vi "Parse Analyzer Results.vi"(6 "Fails":i32[](array[numeric]), 8 "error in":errorcluster, 9 "Passes":i32[](array[numeric]), 10 "VI Paths":path[](array[path]), 11 "Peer Review in":refnum<class "Peer Review.lvclass">) -> (0 "error out":errorcluster, 3 "Peer Review out":refnum<class "Peer Review.lvclass">)   [LabVIEW 2020, in "Peer Review.lvclass"]
uses:
  Peer Review.lvclass
  <vilib>/Utility/miscctls.llb/LVRowAndColumnUnsignedTypeDef.ctl
  Peer Review.lvclass/Peer Review.ctl
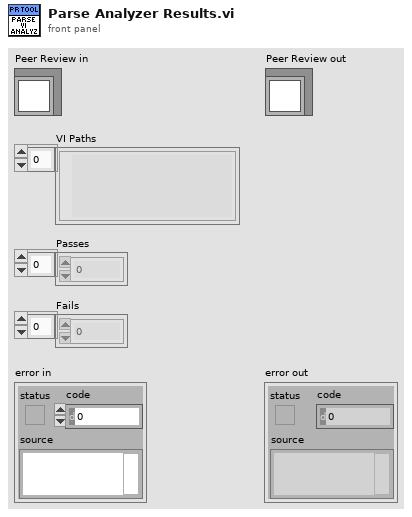
[diagram p1: front panel]
types:
  T1 = typedef "LVRowAndColumnUnsignedTypeDef.ctl" = cluster{"Row":u32, "Column":u32}
  T2 = typedef "Peer Review.lvclass/File Info.ctl" = cluster{"File ID":i32, "Commit ID":i32, "Reviewed Hash":string, "Relative Path":string, "File Path":path, "File Checksum":string, "State":T3, "FP Changes":i32, "BD Changes":i32, "FP Bounds Error":dbl, "BD Bounds Error":dbl, "Lines Added":i32, "Lines Removed":i32, "Analysis Passes":i32, "Analysis Fails":i32, "Attribute Changes":i32, "Reentrancy State":string, "Cyclomatic Complexity":i32, "Node Count":i32, "Revision Number":u32, "LabVIEW Version":string, "Description":string, "Master Path":path, "Master Checksum":string, "VI Type":T4, "LabVIEW File":bool, "Review Complete":bool, "File Ref":refnum<vi>}
  T3 = typedef "Peer Review.lvclass/File State.ctl" = enum16{"Interrogation Needed", "Modified", "Deleted", "Added", "Matches Previous", "No Changes", "Moved"}
  T4 = typedef "Peer Review.lvclass/VI Type.ctl" = enum32{"invalid VI type", "Standard VI", "Control VI", "Global VI", "Polymorphic VI", "Configuration VI", "SubSystem", "Facade VI", "Method VI", "Statechart Diagram VI"}
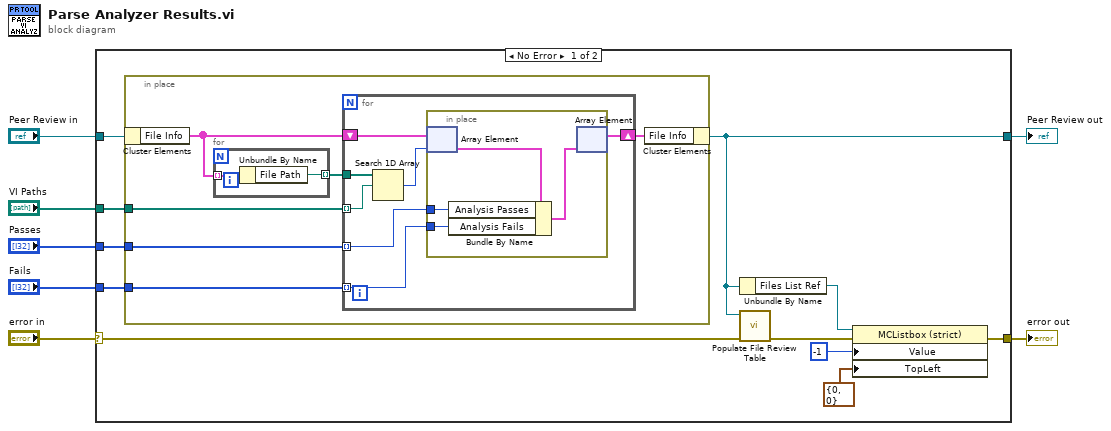
[diagram p0: block diagram]
diagram:
  n1 = case shown="No Error" "error in" {
    selector: "error in" -> [w18 w39]
    tunnel: [w14 w39] -> w6
    tunnel: [w8 w38] -> w4
    tunnel: "Peer Review in" -> [w9 w38]
    tunnel: "VI Paths" -> [w13 _]
    tunnel: "Passes" -> [w12 _]
    tunnel: "Fails" -> [w11 _]
    frame No Error {
      n2 = in-place {
        in-place-border: w13 -> [w23]
        in-place-border: w12 -> [w22]
        in-place-border: w11 -> [w21]
        n3 = in-place-cluster #1(w9) -> ("File Info"=w20:T2[])
        n4 = for {
          tunnel: w20 -> [w26] mode=indexing
          tunnel: [w25] -> w24 mode=indexing
          n5 = Unbundle By Name(w26) -> ("File Path"=w25:path)
        }
        n6 = for {
          tunnel: w24 -> [w33]
          shift-right: [w30] -> w19
          shift-left: w20 -> [w32]
          tunnel: w23 -> [w29] mode=indexing
          tunnel: w22 -> [w28] mode=indexing
          tunnel: w21 -> [w27] mode=indexing
          n7 = Search 1D Array(1D array=w33, element=w29) -> (index of element=w31:i32)  [unwired: 1 in]
          n8 = in-place "In Place Element Structure" {
            in-place-border: w28 -> [w36]
            in-place-border: w27 -> [w35]
            n9 = in-place-array #2(w32, w31) -> (w37:T2)
            n10 = Bundle By Name(cluster=w37, "Analysis Passes"=w36, "Analysis Fails"=w35) -> (w34:T2)
            n11 = in-place-array #2(w34) -> (w30:T2[])  [unwired: 1 out]
          }
        }
        n12 = in-place-cluster #1("File Info"=w19) -> (w8:refnum<class "Peer Review.lvclass">)
      }
      n13 = Unbundle By Name(w8) -> ("Files List Ref"=w10:refnum<vi>)
      n14 = call "Populate File Review Table.vi"("error in"=w18, "Peer Review"=w8) -> ("error out"=w15:errorcluster)  [unwired: 9 in]
      n15 = property on="Property Node" class="MCListbox (strict)"(reference=w10, error in=w15, "Value"=-1, "TopLeft"=T1 {"Row"=0, "Column"=0} ("Top Left Visible Cell")) -> (error out=w14:errorcluster)  [unwired: 1 out]
    }
    frame Error {
    }
  }
  "error out" <- w6
  "Peer Review out" <- w4
